vi "LIDAR V2.5 FPGA Main.vi"() -> ()   [LabVIEW 2013]
uses:
  <vilib>/Platform/TimedLoop/XDataNode/wakeup.ctl
  <vilib>/Platform/TimedLoop/XDataNode/XDNodeRunTimeDep.lvlib
  <vilib>/Platform/TimedLoop/XDataNode/nitl_modes.ctl
  <vilib>/Platform/TimedLoop/XDataNode/timing_clust.ctl
  <vilib>/Platform/TimedLoop/XDataNode/XDataNode.xnode
  <vilib>/rvi/DataTransferAndStorage/Container/XNode/niFpgaContainer.xnode
  <vilib>/rvi/FIFO/Fifo_Resource/nirvififoEmulationWrite.vi
  <vilib>/eio/EIONode/EIONode.xnode
  <vilib>/rvi/eio/common/nirviEmuTemplateMethod_errors.vi
  <vilib>/rvi/FIFO/Fifo_Resource/nirvififoEmulationRead.vi
  Controls/FPGA Nain State.ctl
  LIDAR V2 Globals.vi
  Controls/Algorithm State.ctl
  <vilib>/rvi/interface/RandomDataEmulation/nirviRandomDataFpgaReadWriteTemplate.vi
  Controls/Scan Format Typedaf.ctl
panel:
  out "Sync":bool
  in  "MaxStartSample":u8
  in  "LedScanDebEn":bool
  in  "ActiveLedIndexDeb":u16
  in  "10thIndexDeb":u8
  in  "PulseUpClck":u16=3
  in  "PulseWaitClck":u16=40
  in  "AO Trig":bool
  in  "Devider":u8=3
  in  "PFI3":bool
  in  "PFI2":bool
  in  "User Command Commit":bool
  in  "User Command":u8
  out "User Command Idle":bool
  out "User Command Status":u8
  in  "User Data 0":u8
  in  "User Data 1":u8
  out "User Error":bool
  out "Configured?":bool
  in  "MemDebStart":u32
  in  "MemDebEnd":u32
  in  "ReadMemSel":bool
  in  "ReadMem":bool
  in  "NextLedEn":bool
  out "SimOut":i16
  out "PLL Locked":bool
  out "LedAddress":u16
  in  "SingleCycle":bool
  in  "PulsePerLed":i16=199
  in  "ScanFormat":T1=enum."FullScanPerLed"
  in  "SamplingEnable":bool
  out "MainState":T2
  out "10thIndex":u8
  out "PulseIndex":i16
  in  "MemSel":bool
  in  "ActiveLedIndex":u16
  out "InitMem":bool
  out "PulseEnd":bool
  in  "SampPerPulse":u16=99
  out "IterReset":u16 format="%.0b"
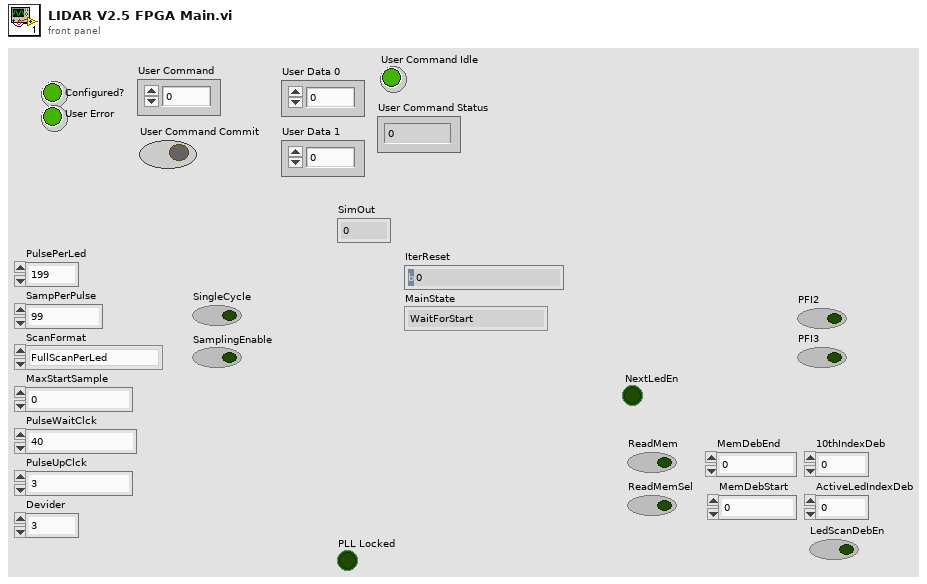
[diagram p1: front panel]
types:
  T1 = typedef "Scan Format Typedaf.ctl" = enum16{"1PulsePerLed", "FullScanPerLed"}
  T2 = typedef "FPGA Nain State.ctl" = enum16{"WaitForStart", "SetProcParams", "SelectActiveLed", "WaitForPulseGenEnd", "ActivatePulse", "WaitForPulseEnd", "WaitForAlgoStart", "SingleCycleEnd"}
  T3 = typedef "XDNodeRunTimeDep.lvlib/timing_clust.ctl" = cluster{"Expected End [f-1]":u64, "Actual End [f-1]":u64, "Finished Late? [f-1]":bool, "Expected End [i-1]":u64, "Actual End [i-1]":u64, "Finished Late? [i-1]":bool, "Expected Start [i]":u64, "Actual Start [i]":u64, "Expected Start [f]":u64, "Actual Start [f]":u64, "Source Name":string, "Structure Name":string, "Period":i64, "Deadline":i64, "Offset":i64, "Start":i64, "Priority":i32, "Timeout":i32, "Mode":T4, "Wakeup Reason":T5, "Error":errorcluster, "Source Type":string, "Secondary Source Type":string, "Global End Time":u64, "Global Start Time":u64, "Frame Duration":u64, "Iteration Duration":u64, "Assigned CPU":i32, "I/O Scan Engine Mode":u32}
  T4 = typedef "XDNodeRunTimeDep.lvlib/nitl_modes.ctl" = enum32{"No Change", "Process missed periods, maintain original phase", "Discard missed periods, maintain original phase", "Process missed periods, ignore original phase", "Discard missed periods, ignore original phase"}
  T5 = typedef "XDNodeRunTimeDep.lvlib/wakeup.ctl" = enum32{"Normal", "Aborted", "Asynchronous wakeup", "Timing source error", "Timed loop error", "Timeout"}
  T6 = typedef "Algorithm State.ctl" = enum16{"WaitForStart", "GetNextSignalElement", "WaitForNextSignalElem", "MultWithSinc", "CalcMax"}
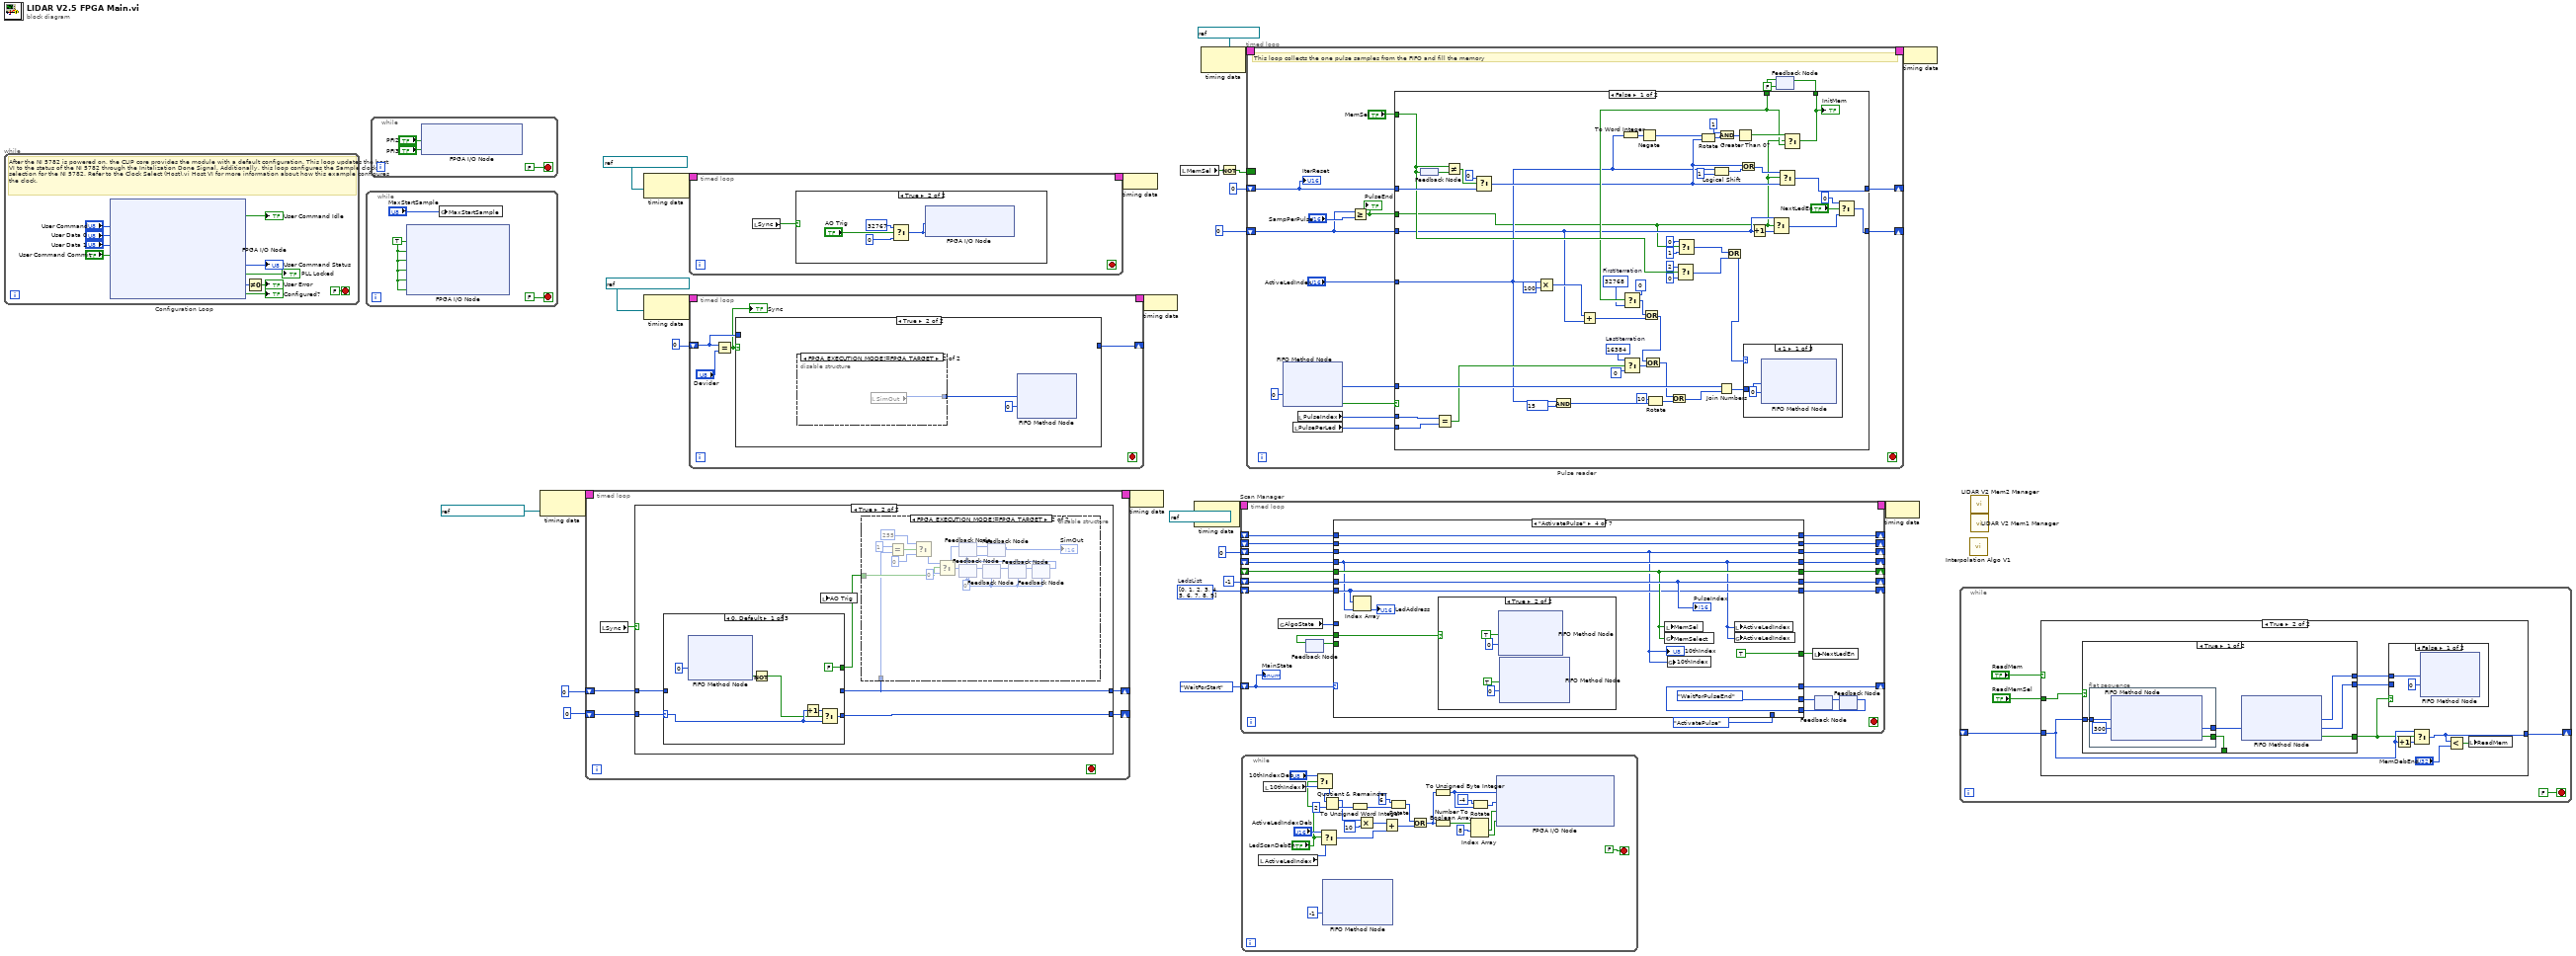
[diagram p0: block diagram]
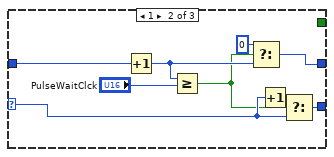
[diagram p5: hidden frame]
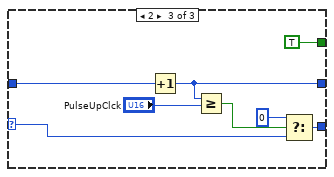
[diagram p6: hidden frame]
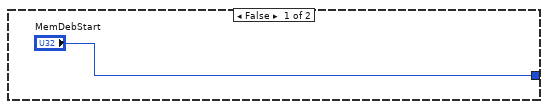
[diagram p7: hidden frame]
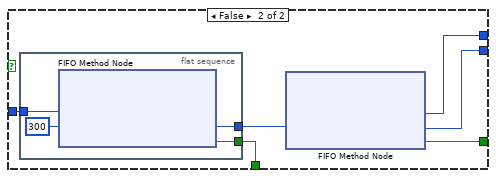
[diagram p9: hidden frame]
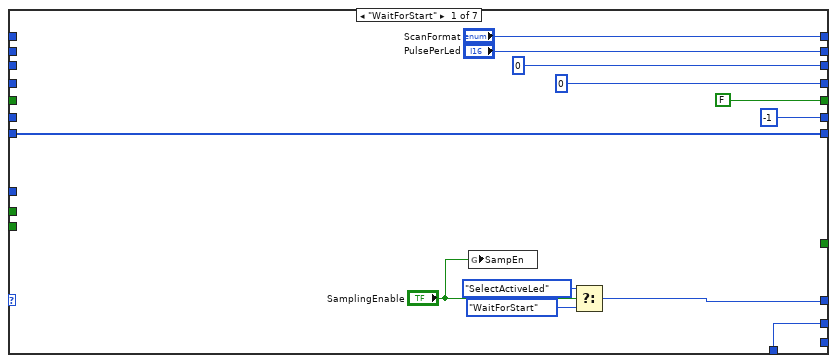
[diagram p10: hidden frame]
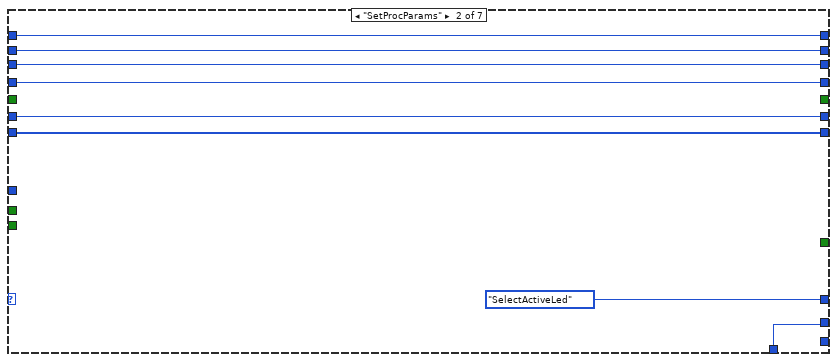
[diagram p11: hidden frame]
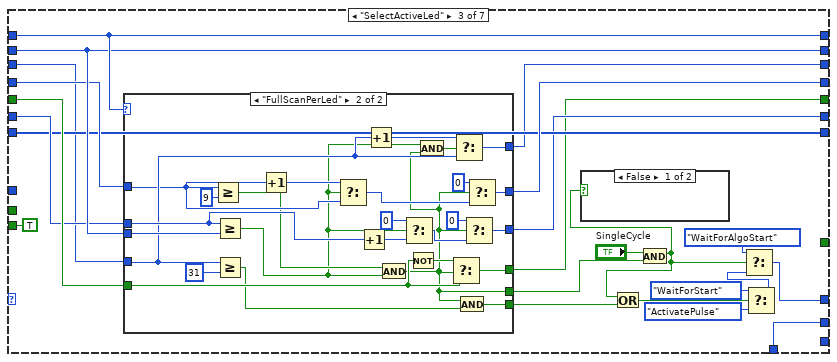
[diagram p12: hidden frame]
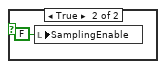
[diagram p13: hidden frame]
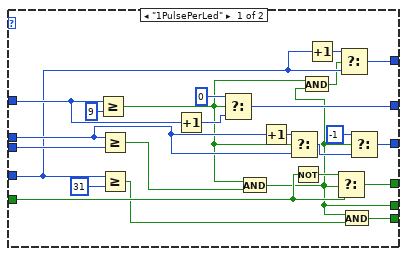
[diagram p14: hidden frame]
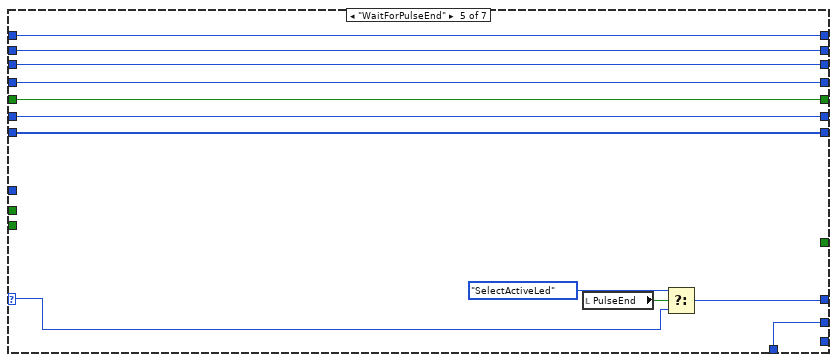
[diagram p16: hidden frame]
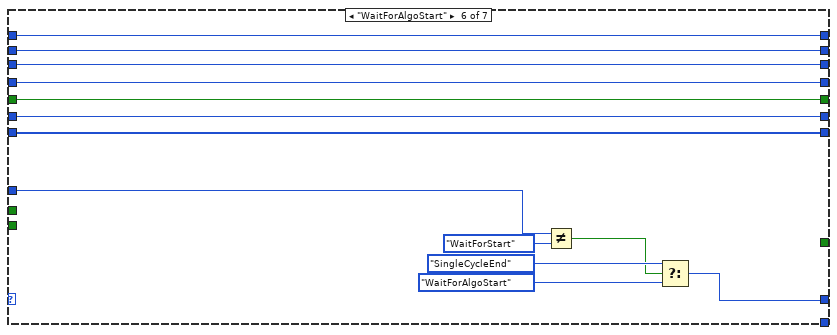
[diagram p17: hidden frame]
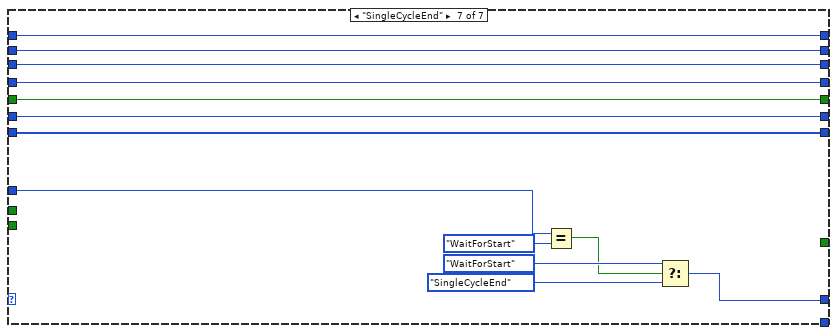
[diagram p18: hidden frame]
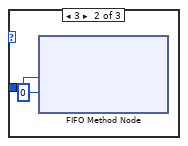
[diagram p19: hidden frame]
diagram:
  w14 = u16[] [0, 1, 2, 3, 4, 5, 6, 7, 8, 9]  # LedsList
  n1 = while "Configuration Loop" {
    stop <- FALSE stop-if-true
    # "After the NI 5782 is powered on, the CLIP core provides the module with a default configuration. This loop updates the host VI to the status of the NI 5782 through the Initalization Done Signal. Additionally, this loop configures the Sample clock selection for the NI 5782. Refer to the Clock Select (Host).vi Host VI for more information about how this example configures the clock."
    n2 = xnode "FPGA I/O Node"("IO Module\\User Command"="User Command", "IO Module\\User Data 0"="User Data 0", "IO Module\\User Data 1"="User Data 1", "IO Module\\User Command Commit"="User Command Commit") -> ("IO Module\\User Command Idle"=→"User Command Idle":bool, "IO Module\\User Command Status"=→"User Command Status":u8, "IO Module\\PLL Locked"=→"PLL Locked":bool, "IO Module\\User Error"=w31:u8, "IO Module\\Initialization Done"=→"Configured?":bool)  [unwired: 9 in, 9 out]
    n3 = Not Equal To 0?(x=w31) -> (x != 0?=→"User Error":bool)
  }
  n4 = while {
    stop <- FALSE stop-if-true
    w39 = TRUE ("IO Module\\DIO Port 0 WE")
    n5 = xnode "FPGA I/O Node"("IO Module\\DIO Port 0 WE"=w39, "IO Module\\DIO Port 1 WE"=w39, "IO Module\\PFI 0 WE"=w39, "IO Module\\PFI 1 WE"=w39, "IO Module\\PFI 2 WE"=w39, "IO Module\\PFI 3 WE"=w39) -> ()  [unwired: 6 in, 6 out]
    n6 = global write "LIDAR V2 Globals.vi" "MaxStartSample"("MaxStartSample") -> ()
  }
  n7 = while {
    stop <- FALSE stop-if-true
    n8 = xnode "FPGA I/O Node"("IO Module\\PFI 2 Wr Data"="PFI2", "IO Module\\PFI 3 Wr Data"="PFI3") -> ()  [unwired: 2 in, 2 out]
  }
  n9 = node-c288(refnum<k21> "IO Module\\Data Clock" ("Source Name")) -> (w8:T3)
  n10 = timed-loop {
    timing: w8 -> [_]
    timing-out: [_] -> w7
    shift-right: [w47] -> _
    shift-left: i16 0 -> [w48]
    shift-right: [w45] -> _
    shift-left: u16 0 -> [w46]
    stop <- _ stop-if-true
    n11 = local read "Sync"() -> (w44:bool)
    n12 = case shown="True" w44 {
      tunnel: w48 -> [w50 w55]
      tunnel: [w50 w54] -> w47
      tunnel: w46 -> [w49 w53]
      tunnel: [w49 w52] -> w45
      frame False {
      }
      frame True {
        n13 = case shown="0, Default" w55 {
          selector: w55 -> [w77 w84 w90]
          tunnel: [w78 w85 w91] -> w54
          tunnel: w53 -> [_ w87 w95]
          tunnel: [_ w81 w94] -> w52
          tunnel: [FALSE _ TRUE] -> w51
          frame 0, Default {
            n14 = xnode ("FIFO Method Node")("Timeout"=0) -> ("Timed Out?"=w74:bool)  [unwired: 1 in, 2 out]
            n15 = Not(x=w74) -> (.not. x?=w72:bool)
            n16 = Increment(x=w77) -> (x+1=w76:i16)
            n17 = Select(t=w76, s=w72, f=w77) -> (s? t:f=w78:i16)
          }
          frame 1 {
            n18 = Increment(x=w87) -> (x+1=w82:u16)
            n19 = Greater Or Equal?(x=w82, y="PulseWaitClck") -> (x >= y?=w79:bool)
            n20 = Select(t=u16 0, s=w79, f=w82) -> (s? t:f=w81:u16)
            n21 = Increment(x=w84) -> (x+1=w83:i16)
            n22 = Select(t=w83, s=w79, f=w84) -> (s? t:f=w85:i16)
          }
          frame 2 {
            n23 = Increment(x=w95) -> (x+1=w94:u16)
            n24 = Greater Or Equal?(x=w94, y="PulseUpClck") -> (x >= y?=w92:bool)
            n25 = Select(t=i16 0, s=w92, f=w90) -> (s? t:f=w91:i16)
          }
        }
        n26 = local write "AO Trig"(w51) -> ()
        n27 = disable-structure shown="FPGA_EXECUTION_MODE!=FPGA_TARGET" {
          disable-tunnel: w51 -> [_ w63]
          disable-tunnel: w52 -> [_ w62]
          frame condition #0 (active) {
          }
          frame condition #1 {
            w66 = i16 0 ("IO Module\\AO 0")
            n28 = Equal?(x=u16 1, y=w62) -> (x = y?=w60:bool)
            n29 = Select(t=i16 255 ("IO Module\\AO 0"), s=w60, f=i16 0) -> (s? t:f=w61:i16)
            n30 = Select(t=w61, s=w63, f=i16 0 ("IO Module\\AO 0")) -> (s? t:f=w64:i16)
            n31 = feedback-in #1(w64) -> ()
            n32 = feedback #1(w66) -> (w71:i16)
            n33 = feedback #2(w66) -> (w67:i16)
            n34 = feedback #3(w66) -> (w70:i16)
            n35 = feedback-in #3(w71) -> ()
            n36 = feedback #4(w66) -> (→"SimOut":i16)
            n37 = feedback-in #4(w67) -> ()
            n38 = feedback #5(w66) -> (w69:i16)
            n39 = feedback-in #5(w70) -> ()
            n40 = feedback #6(w66) -> (w68:i16)
            n41 = feedback-in #2(w68) -> ()
            n42 = feedback-in #6(w69) -> ()
          }
        }
      }
    }
  }
  n43 = node-c288(refnum<k21> "IO Module\\Data Clock" ("Source Name")) -> (w3:T3)
  n44 = node-c288(refnum<k21> "IO Module\\Data Clock" ("Source Name")) -> (w26:T3)
  n45 = timed-loop {
    timing: w3 -> [_]
    timing-out: [_] -> w2
    stop <- _ stop-if-true
    n46 = local read "Sync"() -> (w98:bool)
    n47 = case shown="True" w98 {
      frame False {
      }
      frame True {
        n48 = Select(t=i16 32767 ("IO Module\\AO 0"), s="AO Trig", f=i16 0 ("IO Module\\AO 0")) -> (s? t:f=w99:i16)
        n49 = xnode "FPGA I/O Node"("IO Module\\AO 0 N-1"=w99, "IO Module\\AO 0 N"=w99) -> ()  [unwired: 2 in, 2 out]
      }
    }
  }
  n50 = timed-loop {
    timing: w26 -> [_]
    timing-out: [_] -> w25
    shift-right: [w106] -> _
    shift-left: u8 0 -> [w107]
    stop <- _ stop-if-true
    n51 = Equal?(x=w107, y="Devider") -> (x = y?=w105:bool)
    "Sync" <- w105
    n52 = case shown="True" w105 {
      tunnel: w107 -> [w110 _]
      tunnel: [w109 _] -> w106
      frame False {
        n53 = Increment(x=w110) -> (x+1=w109:u8)
      }
      frame True {
        n54 = disable-structure shown="FPGA_EXECUTION_MODE!=FPGA_TARGET" {
          disable-tunnel: [w113 w114] -> w111
          frame condition #0 (active) {
            n55 = xnode "FPGA I/O Node"() -> ("IO Module\\AI 0"=w113:i16)  [unwired: 1 in, 1 out]
          }
          frame condition #1 {
            n56 = local read "SimOut"() -> (w114:i16)
          }
        }
        n57 = xnode ("FIFO Method Node")("Element"=w111, "Timeout"=0) -> ()  [unwired: 1 in, 2 out]
      }
    }
  }
  n58 = node-c288(w2) -> ()
  n59 = node-c288(w7) -> ()
  n60 = node-c288(w25) -> ()
  n61 = local read "MemSel"() -> (w19:bool)
  n62 = node-c288(refnum<k21> "100 MHz Clock" ("Source Name")) -> (w22:T3)
  n63 = node-c288(refnum<k21> "100 MHz Clock" ("Source Name")) -> (w24:T3)
  n64 = Not(x=w19) -> (.not. x?=w18:bool)
  n65 = timed-loop "Scan Manager" {
    timing: w22 -> [_]
    timing-out: [_] -> w21
    shift-right: [w139] -> _
    shift-left: FPGA_Nain_State."WaitForStart" ("MainState") -> [w140]
    shift-right: [w138] -> _
    shift-left: _ -> [w136]
    shift-right: [w137] -> _
    shift-left: _ -> [w135]
    shift-right: [w128] -> _
    shift-left: u8 0 ("10thIndex") -> [w134]
    shift-right: [w118] -> _
    shift-left: _ -> [w133]
    shift-right: [w122] -> _
    shift-left: _ -> [w132]
    shift-right: [w131] -> _
    shift-left: i16 -1 -> [w121]
    shift-right: [w129] -> _
    shift-left: w14 -> [w130]
    stop <- _ stop-if-true
    n66 = global read "LIDAR V2 Globals.vi" "AlgoState"() -> (w117:T6)
    n67 = feedback #7() -> (w119:bool)  [unwired: 1 in]
    n68 = feedback #8() -> (w125:T2)  [unwired: 1 in]
    n69 = feedback #9() -> (w124:T2)  [unwired: 1 in]
    n70 = case shown="\"ActivatePulse\"" w140 {
      selector: w140 -> [_ _ _ _ w256 _ _]
      tunnel: [w150 FPGA_Nain_State."SelectActiveLed" ("MainState") w164 w242 w255 w266 w279] -> w139
      tunnel: ["ScanFormat" w156 w183 w246 w262 w275 w288] -> w138
      tunnel: ["PulsePerLed" w155 w181 w245 w261 w274 w287] -> w137
      tunnel: w136 -> [_ w156 w183 w246 w262 w275 w288]
      tunnel: w135 -> [_ w155 w181 w245 w261 w274 w287]
      tunnel: [u8 0 ("10thIndex") w154 w172 w235 w260 w273 w286] -> w128
      tunnel: w134 -> [_ w154 w173 w235 w260 w273 w286]
      tunnel: [u16 0 ("ActiveLedIndex") w153 w178 w236 w259 w272 w285] -> w118
      tunnel: w133 -> [_ w153 w179 w236 w259 w272 w285]
      tunnel: [FALSE _ w175 w239 w258 w271 w284] -> w122
      tunnel: w132 -> [_ _ w182 w239 w258 w271 w284]
      tunnel: [i16 -1 ("t") w159 w176 w240 w253 w270 w283] -> w131
      tunnel: w121 -> [_ w159 w180 w240 w253 w270 w283]
      tunnel: w130 -> [w148 w158 w177 w237 w252 w269 w282]
      tunnel: [w148 w158 w177 w237 w252 w269 w282] -> w129
      tunnel: [_ _ _ TRUE ("SampEnable") _ _ _] -> w127
      tunnel: [w147 w157 w171 FPGA_Nain_State."WaitForPulseEnd" ("MainState") w251 _ _] -> w126
      tunnel: w124 -> [_ _ _ w242 _ _ _]
      tunnel: FPGA_Nain_State."ActivatePulse" ("MainState") -> [w147 w157 w171 _ w251 _ _]
      tunnel: [_ _ TRUE _ _ _ _] -> w120
      tunnel: w119 -> [_ _ _ w241 _ _ _]
      tunnel: w117 -> [_ _ _ _ _ w263 w277]
      frame "WaitForStart" {
        n71 = global write "LIDAR V2 Globals.vi" "SampEn"("SamplingEnable") -> ()
        n72 = Select(t=FPGA_Nain_State."SelectActiveLed" ("MainState"), s="SamplingEnable", f=FPGA_Nain_State."WaitForStart" ("MainState")) -> (s? t:f=w150:T2)
      }
      frame "SetProcParams" {
      }
      frame "SelectActiveLed" {
        n73 = case shown="\"FullScanPerLed\"" w183 {
          tunnel: w182 -> [w200 w230]
          tunnel: w173 -> [w193 w225]
          tunnel: w181 -> [w203 w232]
          tunnel: w179 -> [w206 w216]
          tunnel: w180 -> [w202 w231]
          tunnel: [w194 w212] -> w178
          tunnel: [w189 w214] -> w176
          tunnel: [w197 w228] -> w175
          tunnel: [w195 w226] -> w169
          tunnel: [w191 w223] -> w172
          tunnel: [w185 w209] -> w170
          frame "1PulsePerLed" {
            n74 = Greater Or Equal?(x=w206, y=u16 9) -> (x >= y?=w187:bool)
            n75 = Greater Or Equal?(x=w202, y=w203) -> (x >= y?=w198:bool)
            n76 = Greater Or Equal?(x=w193, y=u8 31) -> (x >= y?=w196:bool)
            n77 = Increment(x=w206) -> (x+1=w205:u16)
            n78 = Select(t=u16 0, s=w187, f=w205) -> (s? t:f=w194:u16)
            n79 = And(x=w187, y=w198) -> (x .and. y?=w185:bool)
            n80 = Increment(x=w202) -> (x+1=w201:i16)
            n81 = Select(t=w201, s=w187, f=w202) -> (s? t:f=w190:i16)
            n82 = Not(x=w200) -> (.not. x?=w199:bool)
            n83 = And(x=w187, y=w185) -> (x .and. y?=w186:bool)
            n84 = Increment(x=w193) -> (x+1=w192:u8)
            n85 = Select(t=w199, s=w185, f=w200) -> (s? t:f=w197:bool)
            n86 = Select(t=w192, s=w186, f=w193) -> (s? t:f=w191:u8)
            n87 = And(x=w185, y=w196) -> (x .and. y?=w195:bool)
            n88 = Select(t=i16 -1, s=w185, f=w190) -> (s? t:f=w189:i16)
          }
          frame "FullScanPerLed" {
            n89 = Greater Or Equal?(x=w216, y=u16 9) -> (x >= y?=w215:bool)
            n90 = Greater Or Equal?(x=w231, y=w232) -> (x >= y?=w210:bool)
            n91 = Greater Or Equal?(x=w225, y=u8 31) -> (x >= y?=w227:bool)
            n92 = Increment(x=w216) -> (x+1=w217:u16)
            n93 = Select(t=w217, s=w210, f=w216) -> (s? t:f=w213:u16)
            n94 = Increment(x=w231) -> (x+1=w219:i16)
            n95 = Increment(x=w225) -> (x+1=w224:u8)
            n96 = And(x=w215, y=w210) -> (x .and. y?=w209:bool)
            n97 = Select(t=i16 0, s=w210, f=w219) -> (s? t:f=w222:i16)
            n98 = Not(x=w230) -> (.not. x?=w229:bool)
            n99 = And(x=w210, y=w209) -> (x .and. y?=w220:bool)
            n100 = Select(t=w229, s=w209, f=w230) -> (s? t:f=w228:bool)
            n101 = Select(t=w224, s=w220, f=w225) -> (s? t:f=w223:u8)
            n102 = And(x=w209, y=w227) -> (x .and. y?=w226:bool)
            n103 = Select(t=i16 0, s=w209, f=w222) -> (s? t:f=w214:i16)
            n104 = Select(t=u16 0, s=w209, f=w213) -> (s? t:f=w212:u16)
          }
        }
        n105 = And(x="SingleCycle", y=w170) -> (x .and. y?=w161:bool)
        n106 = case shown="False" w161 {
          frame False {
          }
          frame True {
            n107 = local write "SamplingEnable"(FALSE ("SamplingEnable")) -> ()
          }
        }
        n108 = Or(x=w161, y=w169) -> (x .or. y?=w168:bool)
        n109 = Select(t=FPGA_Nain_State."WaitForStart" ("MainState"), s=w168, f=FPGA_Nain_State."ActivatePulse" ("MainState")) -> (s? t:f=w165:T2)
        n110 = Select(t=FPGA_Nain_State."WaitForAlgoStart" ("MainState"), s=w161, f=w165) -> (s? t:f=w164:T2)
      }
      frame "ActivatePulse" {
        n111 = Index Array(array=w237, index=w236) -> (element=→"LedAddress":u16)
        n112 = case shown="True" w241 {
          frame False {
          }
          frame True {
            n113 = xnode ("FIFO Method Node")("Element"=TRUE ("GenPulse"), "Timeout"=0) -> ()  [unwired: 1 in, 2 out]
            n114 = xnode ("FIFO Method Node")("Element"=TRUE ("GenPulse"), "Timeout"=0) -> ()  [unwired: 1 in, 2 out]
          }
        }
        n115 = local write "MemSel"(w239) -> ()
        n116 = global write "LIDAR V2 Globals.vi" "MemSelect"(w239) -> ()
        n117 = global write "LIDAR V2 Globals.vi" "10thIndex"(w235) -> ()
        n118 = local write "ActiveLedIndex"(w236) -> ()
        n119 = global write "LIDAR V2 Globals.vi" "ActiveLedIndex"(w236) -> ()
        "PulseIndex" <- w240
        "10thIndex" <- w235
      }
      frame "WaitForPulseEnd" {
        n120 = local read "PulseEnd"() -> (w257:bool)
        n121 = Select(t=FPGA_Nain_State."SelectActiveLed", s=w257, f=w256) -> (s? t:f=w255:T2)
      }
      frame "WaitForAlgoStart" {
        n122 = Not Equal?(x=w263, y=Algorithm_State."WaitForStart") -> (x != y?=w264:bool)
        n123 = Select(t=FPGA_Nain_State."SingleCycleEnd", s=w264, f=FPGA_Nain_State."WaitForAlgoStart" ("MainState")) -> (s? t:f=w266:T2)
      }
      frame "SingleCycleEnd" {
        n124 = Equal?(x=w277, y=Algorithm_State."WaitForStart") -> (x = y?=w276:bool)
        n125 = Select(t=FPGA_Nain_State."WaitForStart", s=w276, f=FPGA_Nain_State."SingleCycleEnd" ("MainState")) -> (s? t:f=w279:T2)
      }
    }
    n126 = feedback-in #7(w120) -> ()
    n127 = local write "NextLedEn"(w127) -> ()
    n128 = feedback-in #8(w126) -> ()
    n129 = feedback-in #9(w125) -> ()
    "MainState" <- w140
  }
  n130 = while {
    stop <- FALSE stop-if-true
    n131 = local read "ActiveLedIndex"() -> (w295:u16)
    n132 = local read "10thIndex"() -> (w297:u8)
    n133 = Select(t="10thIndexDeb", s="LedScanDebEn", f=w297) -> (s? t:f=w296:u8)
    n134 = Select(t="ActiveLedIndexDeb", s="LedScanDebEn", f=w295) -> (s? t:f=w294:u16)
    n135 = xnode ("FIFO Method Node")("Timeout"=-1) -> ()  [unwired: 1 in, 3 out]
    n136 = Quotient & Remainder(x=w296, y=u8 2) -> (x-y*floor(x/y)=w301:u8, floor(x/y)=w302:u8)
    n137 = To Unsigned Word Integer(number=w302) -> (unsigned 16bit integer=w309:u16)
    n138 = Multiply(x=w301, y=u8 10) -> (x*y=w300:u8)
    n139 = Add(x=w300, y=w294) -> (x+y=w315:u16)
    n140 = Rotate(1:w309, 2:u16 6 ("x")) -> (0:w316:u16)
    n141 = Or(x=w316, y=w315) -> (x .or. y?=w314:u16)
    n142 = To Unsigned Byte Integer(number=w314) -> (unsigned 8bit integer=w306:u8)
    n143 = Number To Boolean Array(number=w314) -> (Boolean array=w313:bool[])
    n144 = Index Array(array=w313, index #1=8 ("index")) -> (element #1=w311:bool, element #2=w310:bool)  [unwired: 1 in]
    n145 = Rotate(1:w306, 2:i16 -4 ("y")) -> (0:w304:u8)
    n146 = xnode "FPGA I/O Node"("IO Module\\DIO Port 0 Wr Data"=w306, "IO Module\\DIO Port 1 Wr Data"=w304, "IO Module\\PFI 0 Wr Data"=w311, "IO Module\\PFI 1 Wr Data"=w310) -> ()  [unwired: 4 in, 4 out]
  }
  n147 = timed-loop "Pulse reader" {
    timing: w24 -> [_]
    timing-out: [_] -> w23
    shift-right: [w329] -> _
    shift-left: u16 0 -> [w327]
    border: w18 -> [_]
    shift-right: [w320] -> _
    shift-left: u16 0 -> [w318]
    stop <- _ stop-if-true
    # "This loop collects the one pulse samples from the FIFO and fill the memory"
    n148 = xnode ("FIFO Method Node")("Timeout"=0) -> ("Element"=w331:i16, "Timed Out?"=w330:bool)  [unwired: 1 in, 1 out]
    n149 = local read "PulsePerLed"() -> (w321:i16)
    n150 = local read "PulseIndex"() -> (w322:i16)
    n151 = Greater Or Equal?(x=w318, y="SampPerPulse") -> (x >= y?=w317:bool)
    "PulseEnd" <- w317
    n152 = feedback #10(FALSE) -> (w325:bool)
    n153 = case shown="False" w330 {
      tunnel: w331 -> [w382 _]
      tunnel: "ActiveLedIndex" -> [w337 _]
      tunnel: [w362 w393] -> w329
      tunnel: w327 -> [w383 w393]
      tunnel: [w342 w392] -> w326
      tunnel: w325 -> [w341 w392]
      tunnel: "MemSel" -> [w354 _]
      tunnel: w322 -> [w380 _]
      tunnel: w321 -> [w379 _]
      tunnel: [w335 w391] -> w320
      tunnel: w318 -> [w334 w391]
      tunnel: w317 -> [w333 _]
      frame False {
        w372 = u16 16384  # LastIterration
        w339 = u16 32768  # FirstIterration
        n154 = feedback #11() -> (w385:bool)
        n155 = feedback-in #11(w354) -> ()
        n156 = Equal?(x=w380, y=w379) -> (x = y?=w381:bool)
        n157 = Not Equal?(x=w354, y=w385) -> (x != y?=w386:bool)
        n158 = Select(t=u16 0, s=w386, f=w383) -> (s? t:f=w340:u16)
        n159 = Multiply(x=w337, y=u16 100) -> (x*y=w377:u16)
        n160 = And(x=w337, y=u16 15) -> (x .and. y?=w368:u16)
        n161 = Add(x=w377, y=w334) -> (x+y=w376:u16)
        n162 = To Word Integer(number=w337) -> (16bit integer=w348:i16)
        n163 = Select(t=u16 0 ("x"), s=w341, f=w339) -> (s? t:f=w375:u16)
        n164 = Select(t=w372, s=w381, f=u16 0 ("x")) -> (s? t:f=w371:u16)
        n165 = Negate(x=w348) -> (-x=w344:i16)
        n166 = Or(x=w375, y=w376) -> (x .or. y?=w370:u16)
        n167 = Or(x=w370, y=w371) -> (x .or. y?=w365:u16)
        n168 = Rotate(1:w368, 2:i16 10 ("y")) -> (0:w366:u16)
        n169 = Or(x=w365, y=w366) -> (x .or. y?=w364:u16)
        n170 = Select(t=i16 2, s=w354, f=i16 0) -> (s? t:f=w350:i16)
        n171 = Select(t=i16 0, s=w333, f=i16 1) -> (s? t:f=w349:i16)
        n172 = Rotate(1:w340, 2:w344) -> (0:w345:u16)
        n173 = Logical Shift(y=w337, x=u16 1) -> (x << y=w359:u16)
        n174 = Join Numbers(hi=w382, lo=w364) -> ((hi.lo)=w374:u32)
        n175 = And(x=u16 1, y=w345) -> (x .and. y?=w347:u16)
        n176 = Or(x=w349, y=w350) -> (x .or. y?=w351:i16)
        n177 = Greater Than 0?(x=w347) -> (x > 0?=w343:bool)
        n178 = Or(x=w340, y=w359) -> (x .or. y?=w357:u16)
        n179 = case shown="1" w351 {
          tunnel: w374 -> [w387 w389 _]
          frame 1 {
            n180 = xnode ("FIFO Method Node")("Element"=w387, "Timeout"=0) -> ()  [unwired: 1 in, 2 out]
          }
          frame 3 {
            n181 = xnode ("FIFO Method Node")("Element"=w389, "Timeout"=0) -> ()  [unwired: 1 in, 2 out]
          }
          frame Default {
          }
        }
        n182 = Increment(x=w334) -> (x+1=w363:u16)
        n183 = Select(t=w334, s=w333, f=w363) -> (s? t:f=w336:u16)
        n184 = Select(t=w357, s=w333, f=w340) -> (s? t:f=w362:u16)
        n185 = Select(t=w343, s=w333, f=w341) -> (s? t:f=w342:bool)
        "InitMem" <- w342
        n186 = Select(t=u16 0, s="NextLedEn", f=w336) -> (s? t:f=w335:u16)
      }
      frame True {
      }
    }
    n187 = feedback-in #10(w326) -> ()
    "IterReset" <- w327
  }
  n188 = node-c288(w21) -> ()
  n189 = node-c288(w23) -> ()
  n190 = while {
    shift-right: [w398] -> _
    shift-left: _ -> [w397]
    stop <- FALSE stop-if-true
    n191 = case shown="True" "ReadMem" {
      tunnel: "ReadMemSel" -> [_ w405]
      tunnel: ["MemDebStart" w408] -> w398
      tunnel: w397 -> [_ w410]
      frame False {
      }
      frame True {
        n192 = case shown="True" w405 {
          tunnel: w410 -> [w417 w425]
          tunnel: [w416 w424] -> w402
          tunnel: [w415 w423] -> w404
          tunnel: [w414 w422] -> w403
          tunnel: [w413 w421] -> _
          frame True {
            n193 = flat-sequence {
              tunnel: w417 -> [w420]
              tunnel: [w419] -> w414
              tunnel: [w418] -> w413
              frame #0 {
                w419 = 300 ("Timeout")
                n194 = xnode ("FIFO Method Node")("Element"=w420, "Timeout"=w419) -> ("Timed Out?"=w418:bool)  [unwired: 1 in, 1 out]
              }
            }
            n195 = xnode ("FIFO Method Node")("Timeout"=w414) -> ("Element"=w415:u64, "Timed Out?"=w416:bool)  [unwired: 1 in, 1 out]
          }
          frame False {
            n196 = flat-sequence {
              tunnel: w425 -> [w428]
              tunnel: [w427] -> w422
              tunnel: [w426] -> w421
              frame #0 {
                w427 = 300 ("Timeout")
                n197 = xnode ("FIFO Method Node")("Element"=w428, "Timeout"=w427) -> ("Timed Out?"=w426:bool)  [unwired: 1 in, 1 out]
              }
            }
            n198 = xnode ("FIFO Method Node")("Timeout"=w422) -> ("Element"=w423:u64, "Timed Out?"=w424:bool)  [unwired: 1 in, 1 out]
          }
        }
        n199 = case shown="False" w402 {
          tunnel: w404 -> [w412 _]
          tunnel: w403 -> [_ _]
          frame False {
            n200 = xnode ("FIFO Method Node")("Element"=w412, "Timeout"=0) -> ()  [unwired: 1 in, 2 out]
          }
          frame True {
          }
        }
        n201 = Increment(x=w410) -> (x+1=w409:u32)
        n202 = Select(t=w410, s=w402, f=w409) -> (s? t:f=w408:u32)
        n203 = Less?(x=w408, y="MemDebEnd") -> (x < y?=w406:bool)
        n204 = local write "ReadMem"(w406) -> ()
      }
    }
  }
  n205 = call "Interpolation Algo V1.vi"() -> ()  [unwired: 10 in, 2 out]
  n206 = call "LIDAR V2 Mem2 Manager.vi"() -> ()  [unwired: 12 in]
  n207 = call "LIDAR V2 Mem1 Manager.vi"() -> ()  [unwired: 12 in]
